vi "LinearAlgebraSub.vi"(9 "C in":fxp<+/-,32,16>[](array[numeric])=[0.0, 0.0, 0.0, 0.0], 10 "B":fxp<+/-,32,16>[](array[numeric])=[0.0, 0.0, 0.0, 0.0], 11 "A":fxp<+/-,32,16>[](array[numeric])=[0.0, 0.0, 0.0, 0.0, 0.0, 0.0, 0.0, 0.0, 0.0, 0.0, 0.0, 0.0, 0.0, 0.0, 0.0, 0.0]) -> (2 "C out":fxp<+/-,32,16>[](array[numeric]), 3 "Cycle Count":i32)   [LabVIEW 2025]
uses:
  <vilib>/Platform/TimedLoop/XDataNode/wakeup.ctl
  <vilib>/Platform/TimedLoop/XDataNode/XDNodeRunTimeDep.lvlib
  <vilib>/Platform/TimedLoop/XDataNode/nitl_modes.ctl
  <vilib>/Platform/TimedLoop/XDataNode/timing_clust.ctl
  <vilib>/platform/TimedLoop/XDataNode/XDataNode.xnode
  <vilib>/rvi/linearAlgebra/MatrixMultiply/XNode/nifxpla_MatrixMultiply.xnode
  <vilib>/rvi/linearAlgebra/MatrixMultiply/simVIs/nifxpla_MatrixMultiply_SimTemplateEinEout.vi
  <vilib>/rvi/linearAlgebra/MatrixMultiply/simVIs/nifxpla_MatrixMultiply_SimTemplateEinVout.vi
  <vilib>/rvi/linearAlgebra/MatrixMultiply/simVIs/nifxpla_MatrixMultiply_SimTemplateVinEout.vi
  <vilib>/rvi/linearAlgebra/MatrixMultiply/simVIs/nifxpla_MatrixMultiply_SimTemplateVinVout.vi
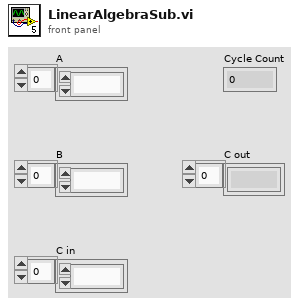
[diagram p1: front panel]
types:
  T1 = typedef "XDNodeRunTimeDep.lvlib/timing_clust.ctl" = cluster{"Expected End [f-1]":u64, "Actual End [f-1]":u64, "Finished Late? [f-1]":bool, "Expected End [i-1]":u64, "Actual End [i-1]":u64, "Finished Late? [i-1]":bool, "Expected Start [i]":u64, "Actual Start [i]":u64, "Expected Start [f]":u64, "Actual Start [f]":u64, "Source Name":string, "Structure Name":string, "Period":i64, "Deadline":i64, "Offset":i64, "Start":i64, "Priority":i32, "Timeout":i32, "Mode":T2, "Wakeup Reason":T3, "Error":errorcluster, "Source Type":string, "Secondary Source Type":string, "Global End Time":u64, "Global Start Time":u64, "Frame Duration":u64, "Iteration Duration":u64, "Assigned CPU":i32, "I/O Scan Engine Mode":u32}
  T2 = typedef "XDNodeRunTimeDep.lvlib/nitl_modes.ctl" = enum32{"No Change", "Process missed periods, maintain original phase", "Discard missed periods, maintain original phase", "Process missed periods, ignore original phase", "Discard missed periods, ignore original phase"}
  T3 = typedef "XDNodeRunTimeDep.lvlib/wakeup.ctl" = enum32{"Normal", "Aborted", "Asynchronous wakeup", "Timing source error", "Timed loop error", "Timeout"}
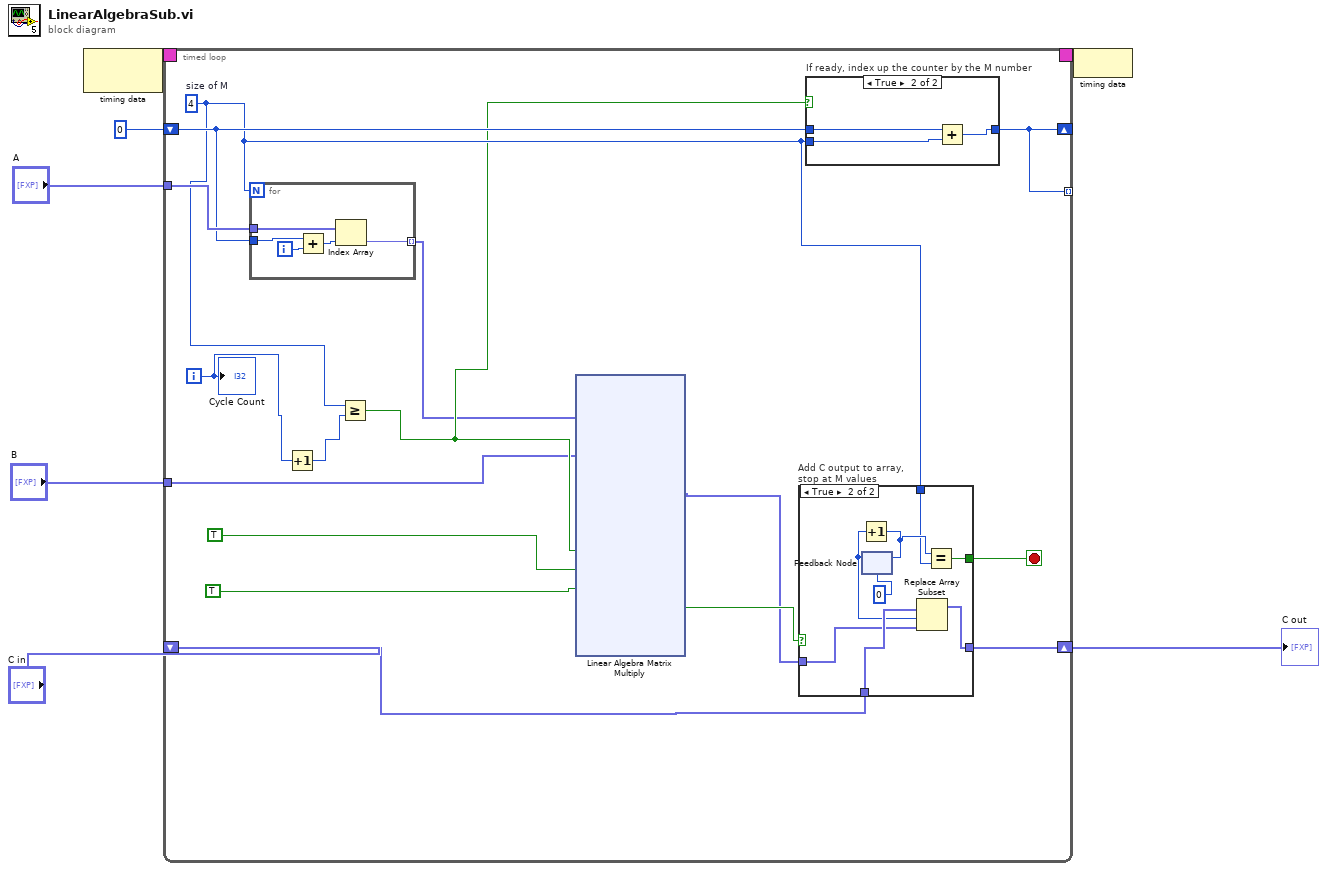
[diagram p0: block diagram]
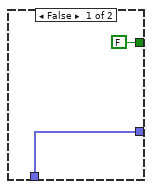
[diagram p3: hidden frame]
diagram:
  n1 = node-c288() -> (w7:T1)  [unwired: 1 in]
  n2 = timed-loop {
    timing: w7 -> [_]
    timing-out: [_] -> w6
    shift-right: [w21] -> w4
    shift-left: "C in" -> [w20]
    tunnel: "B" -> [w9]
    tunnel: "A" -> [w18]
    shift-right: [w15] -> _
    shift-left: 0 ("length") -> [w17]
    tunnel: [w15] -> _ mode=indexing
    i -> [w12]
    stop <- w19 stop-if-true
    w14 = 4  # size of M
    n3 = for {
      N: w14 -> [_]
      tunnel: w18 -> [w28]
      tunnel: w17 -> [w26]
      tunnel: [w24] -> w10 mode=indexing
      i -> [w27]
      n4 = Add(x=w26, y=w27) -> (x+y=w25:i32)
      n5 = Index Array "Index Array"(array=w28, index=w25) -> (element=w24:fxp<+/-,32,16>)
    }
    n6 = Increment(x=w12) -> (x+1=w11:i32)
    n7 = Greater Or Equal?(x=w14, y=w11) -> (x >= y?=w13:bool)
    n8 = xnode ("Linear Algebra Matrix Multiply")("ar"=w10, "br"=w9, "a valid"=w13, "b valid"=TRUE, "ready for output (T)"=TRUE) -> ("cr"=w8:fxp<+/-,32,16>[], "output valid"=w22:bool)  [unwired: 2 in, 4 out]
    n9 = case "Add C output to array, stop at M values" shown="True" w22 {
      tunnel: w8 -> [_ w38]
      tunnel: [w34 w41] -> w21
      tunnel: w20 -> [w34 w42]
      tunnel: [FALSE w39] -> w19
      tunnel: w14 -> [_ w35]
      frame False {
      }
      frame True {
        n10 = feedback #1(0 ("x")) -> (w37:i32)
        n11 = Increment(x=w37) -> (x+1=w36:i32)
        n12 = feedback-in #1(w36) -> ()
        n13 = Replace Array Subset(array=w42, new element=w38, index=w37) -> (w41:fxp<+/-,32,16>[])
        n14 = Equal?(x=w36, y=w35) -> (x = y?=w39:bool)
      }
    }
    n15 = case "If ready, index up the counter by the M number" shown="True" w13 {
      tunnel: w17 -> [w29 w32]
      tunnel: [w29 w31] -> w15
      tunnel: w14 -> [_ w30]
      frame False {
      }
      frame True {
        n16 = Add(x=w32, y=w30) -> (x+y=w31:i32)
      }
    }
    "Cycle Count" <- w12
  }
  "C out" <- w4
  n17 = node-c288(w6) -> ()
